vi "Notifier Actor.vi"(10 "Spawn":refnum<class "Spawn.lvclass">, 11 "Actor in":refnum<class "Actor.lvclass">) -> (0 "Error out":errorcluster, 3 "Actor out":refnum<class "Actor.lvclass">)   [LabVIEW 2025, in "jettl.lvlib" / "Actor.lvclass"]
uses:
  Actor.lvclass
  Spawn/Spawn/Spawn.lvclass
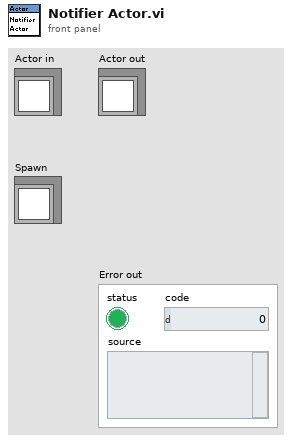
[diagram p1: front panel]
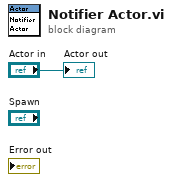
[diagram p0: block diagram]
diagram:
  "Actor out" <- "Actor in"
